vi "Write N attempt.vi"(8 "error in (no error)":errorcluster, 10 "N attempt":i32, 11 "Master CR in":refnum<class "WebSocket Client CR.lvclass">) -> (0 "error out":errorcluster, 3 "Master CR out":refnum<class "WebSocket Client CR.lvclass">)   [LabVIEW 2021, in "WebSockets.lvlib" / "WebSocket Client CR.lvclass"]
uses:
  WebSocket Client CR.lvclass
  WebSocket Client CR.lvclass/WebSocket Client CR.ctl
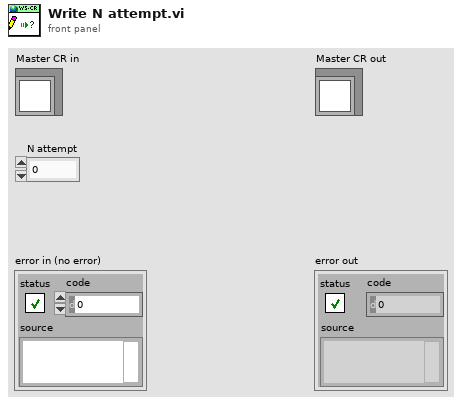
[diagram p1: front panel]
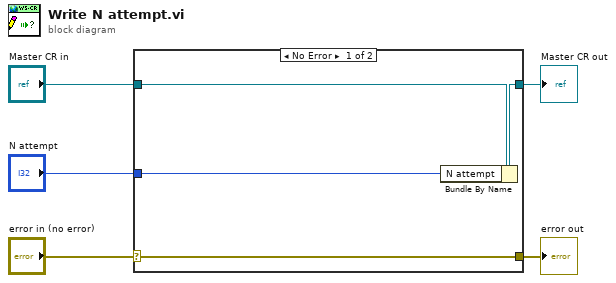
[diagram p0: block diagram]
diagram:
  n1 = case shown="No Error" "error in (no error)" {
    selector: "error in (no error)" -> [w9 w10]
    tunnel: [w9 w10] -> w4
    tunnel: [w7 w11] -> w2
    tunnel: "Master CR in" -> [w8 w11]
    tunnel: "N attempt" -> [w6 _]
    frame No Error {
      n2 = Bundle By Name(cluster=w8, "N attempt"=w6) -> (w7:refnum<class "WebSocket Client CR.lvclass">)
    }
    frame Error {
    }
  }
  "error out" <- w4
  "Master CR out" <- w2
